vi "ShowMatchesTrack.vi"(0 "Refnum in":T2, 5 "Matches (Color Location 3)":T1(array[cluster]), 9 "Color":u32, 11 "error in (no error)":errorcluster) -> (4 "Refnum out":T2, 6 "X1":sgl, 8 "Y1":sgl, 10 "X2":sgl, 14 "error out":errorcluster, 15 "Y2":sgl)   [LabVIEW 2015]
uses:
  <vilib>/vision/Image Controls.llb/IMAQ Image.ctl
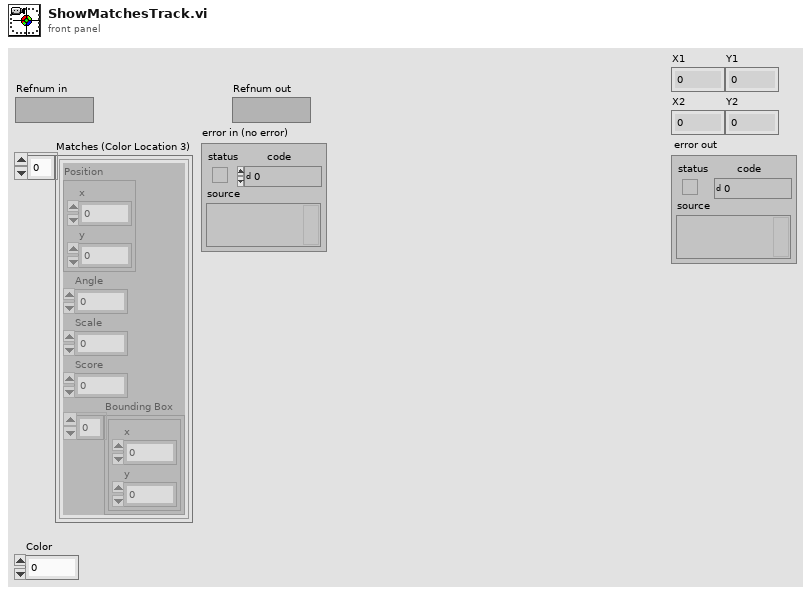
[diagram p1: front panel]
types:
  T1 = cluster{"Position":cluster{"x":sgl, "y":sgl}, "Angle":sgl, "Scale":sgl, "Score":sgl, "Bounding Box":cluster{"x":sgl, "y":sgl}[]}[]
  T2 = typedef "IMAQ Image.ctl" = refnum<image>
  T3 = cluster{"Matches (Color Location 3)[0]":cluster{"Position":cluster{"x":sgl, "y":sgl}, "Angle":sgl, "Scale":sgl, "Score":sgl, "Bounding Box":cluster{"x":sgl, "y":sgl}[]}, "Matches (Color Location 3)[1]":cluster{"Position":cluster{"x":sgl, "y":sgl}, "Angle":sgl, "Scale":sgl, "Score":sgl, "Bounding Box":cluster{"x":sgl, "y":sgl}[]}, "Matches (Color Location 3)[2]":cluster{"Position":cluster{"x":sgl, "y":sgl}, "Angle":sgl, "Scale":sgl, "Score":sgl, "Bounding Box":cluster{"x":sgl, "y":sgl}[]}, "Matches (Color Location 3)[3]":cluster{"Position":cluster{"x":sgl, "y":sgl}, "Angle":sgl, "Scale":sgl, "Score":sgl, "Bounding Box":cluster{"x":sgl, "y":sgl}[]}}
  T4 = cluster{"Bounding Box[0]":cluster{"x":sgl, "y":sgl}, "Bounding Box[1]":cluster{"x":sgl, "y":sgl}, "Bounding Box[2]":cluster{"x":sgl, "y":sgl}, "Bounding Box[3]":cluster{"x":sgl, "y":sgl}}
  T5 = cluster{"[0]":sgl, "[1]":sgl, "[2]":sgl, "[3]":sgl}
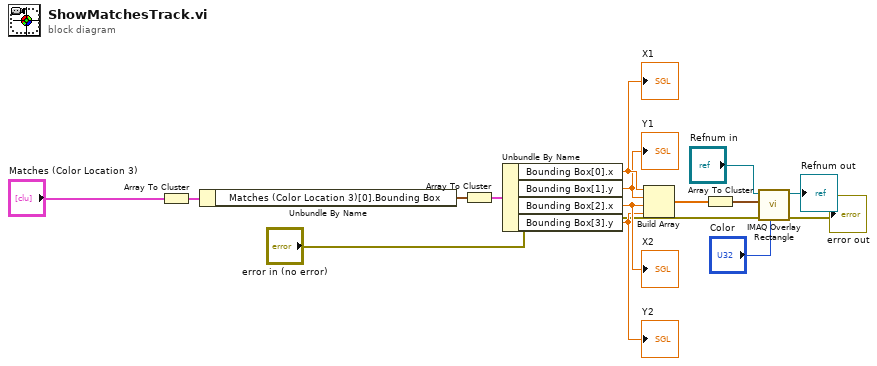
[diagram p0: block diagram]
diagram:
  n1 = Array To Cluster(array="Matches (Color Location 3)") -> (cluster=w10:T3)
  n2 = Unbundle By Name(w10) -> ("Matches (Color Location 3)[0].Bounding Box"=w3:cluster{"x":sgl, "y":sgl}[])
  n3 = Array To Cluster(array=w3) -> (cluster=w4:T4)
  n4 = Unbundle By Name(w4) -> ("Bounding Box[0].x"=w15:sgl, "Bounding Box[1].y"=w7:sgl, "Bounding Box[2].x"=w6:sgl, "Bounding Box[3].y"=w5:sgl)
  "X1" <- w15
  "Y1" <- w7
  "X2" <- w6
  "Y2" <- w5
  n5 = Build Array(w15, w7, w6, w5) -> (w8:sgl[])
  n6 = Array To Cluster(array=w8) -> (cluster=w9:T5)
  n7 = call "IMAQ Overlay Rectangle"("Color"="Color", "error in (no error)"="error in (no error)", "Rectangle"=w9, "Image"="Refnum in") -> ("error out"=→"error out":errorcluster, "Image Out"=→"Refnum out":T2)  [unwired: 6 in]
